vi "Test File IO.vi"() -> ()   [LabVIEW 2013, in "File.lvclass"]
uses:
  File.lvclass
panel:
  out "error out":errorcluster
  in  "New File":bool
  out "spreadsheet string":string
  in  "Write to File":bool
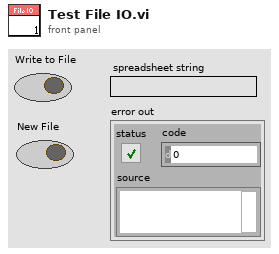
[diagram p1: front panel]
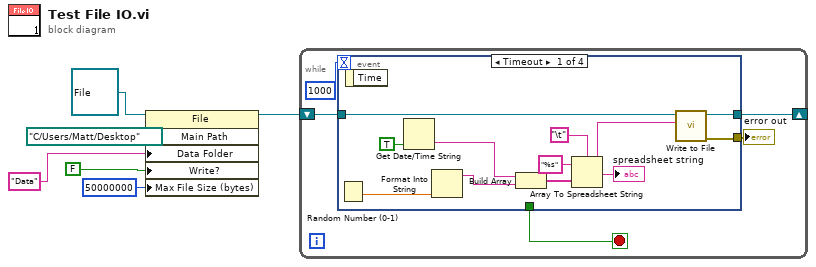
[diagram p0: block diagram]
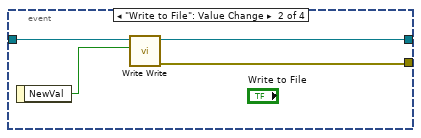
[diagram p2: hidden frame]
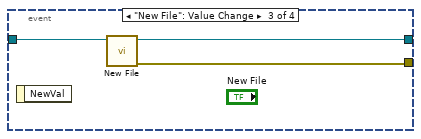
[diagram p3: hidden frame]
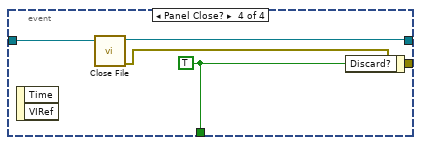
[diagram p4: hidden frame]
diagram:
  n1 = property class="File"(reference=refnum<class "File.lvclass"> refnum ("File"), "Main Path"=path "C:/Users/Matt/Desktop", "Data Folder"="Data", "Write?"=FALSE, "Max File Size (bytes)"=i64 50000000) -> (reference out=w3:refnum<class "File.lvclass">)  [unwired: 1 in, 1 out]
  n2 = while {
    shift-right: [w9] -> _
    shift-left: w3 -> [w11]
    stop <- w8 stop-if-true
    n3 = event shown="[0] Timeout" {
      selector: _ -> [_ _ _ _]
      dyn-events: _ -> [_ _ _ _]
      timeout: 1000 -> [_ _ _ _]
      tunnel: w11 -> [w22 w26 w29 w33]
      tunnel: [w21 w25 w28 w32] -> w9
      tunnel: [_ _ _ w31] -> w8
      tunnel: [w13 w23 w27 w30] -> w7
      event Timeout {
        n4 = Random Number (0-1)() -> (number: 0 to 1=w19:dbl)
        n5 = event-data() -> ()  [unwired: 1 in, 1 out]
        n6 = Get Date/Time String(want seconds? (F)=TRUE) -> (time string=w20:string)  [unwired: 2 in, 1 out]
        n7 = Format Into String(w19) -> (resulting string=w18:string)  [unwired: 3 in, 1 out]
        n8 = Build Array(w20, w18) -> (w17:string[])
        n9 = Array To Spreadsheet String(delimiter (Tab)="\t", array=w17, 3:"%s" ("format string")) -> (spreadsheet string=w16:string)
        "spreadsheet string" <- w16
        n10 = call-dynamic "Write to File.vi"("DataIn"=w16, "File in"=w22) -> ("error out"=w13:errorcluster, "File out"=w21:refnum<class "File.lvclass">)  [unwired: 8 in]
      }
      event "Write to File": Value Change {
        n11 = event-data() -> ("NewVal"=w24:bool)  [unwired: 1 in]
        n12 = call-dynamic "Write Write.vi"("Write?"=w24, "File in"=w26) -> ("error out"=w23:errorcluster, "File out"=w25:refnum<class "File.lvclass">)  [unwired: 8 in]
      }
      event "New File": Value Change {
        n13 = event-data() -> ()  [unwired: 1 in, 1 out]
        n14 = call-dynamic "New File.vi"("File in"=w29) -> ("error out"=w27:errorcluster, "File out"=w28:refnum<class "File.lvclass">)  [unwired: 9 in]
      }
      event Panel Close? {
        w31 = TRUE ("Discard?")
        n15 = event-data() -> ()  [unwired: 1 in, 2 out]
        n16 = call-dynamic "Close File.vi"("File in"=w33) -> ("error out"=w30:errorcluster, "File out"=w32:refnum<class "File.lvclass">)  [unwired: 9 in]
        n17 = event-data("Discard?"=w31) -> ()  [unwired: 1 in, 1 out]
      }
    }
    "error out" <- w7
  }
